vi "Move_to_Start.vi"(5 "Stop":refnum<vi>, 6 "Current Pos":refnum<vi>, 7 "Complete?":refnum<vi>, 8 "Move To":dbl, 9 "error in (no error)":errorcluster, 10 "MG17Motor":refnum<k7>(container)) -> (0 "error out":errorcluster, 2 "reference out":refnum<k7>)   [LabVIEW 2010]
panel:
  in  "#Turns":refnum<vi>
  out "Current":dbl
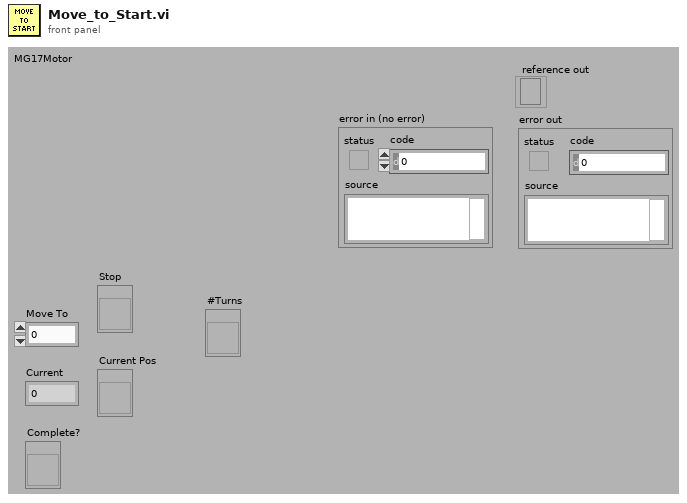
[diagram p1: front panel]
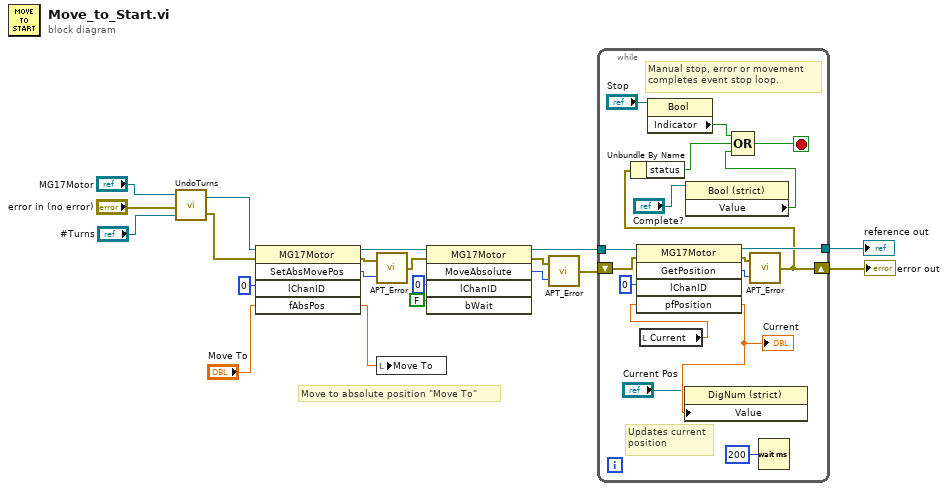
[diagram p0: block diagram]
diagram:
  # "Move to absolute position \"Move To\""
  n1 = call "UndoTurns.vi"("#Turns"="#Turns", "error in (no error)"="error in (no error)", "MG17Motor"="MG17Motor") -> ("error out"=w2:errorcluster, "MG17MotorOut"=w1:refnum<k7>)
  n2 = invoke class="MG17Motor" method="SetAbsMovePos"(reference=w1, error in=w2, "lChanID"=0, "fAbsPos"="Move To") -> (reference out=w6:refnum<k7>, error out=w15:errorcluster, "SetAbsMovePos"=w14:i32, "fAbsPos"=w18:sgl)  [unwired: 1 in, 1 out]
  n3 = call "APT_Error.vi"("Return Code"=w14, "error in (no error)"=w15) -> ("error out"=w13:errorcluster)
  n4 = local write "Move To"(w18) -> ()
  n5 = invoke class="MG17Motor" method="MoveAbsolute"(reference=w6, error in=w13, "lChanID"=0, "bWait"=FALSE) -> (reference out=w9:refnum<k7>, error out=w12:errorcluster, "MoveAbsolute"=w11:i32)  [unwired: 1 in, 2 out]
  n6 = call "APT_Error.vi"("Return Code"=w11, "error in (no error)"=w12) -> ("error out"=w10:errorcluster)
  n7 = while {
    shift-right: [w30] -> w8
    shift-left: w10 -> [w33]
    tunnel: w9 -> [w35]
    tunnel: [w34] -> w7
    stop <- w28 stop-if-true
    # "Updates current\nposition"
    # "Manual stop, error or movement\ncompletes event stop loop."
    n8 = local read "Current"() -> (w26:dbl)
    n9 = invoke class="MG17Motor" method="GetPosition"(reference=w35, error in=w33, "lChanID"=0, "pfPosition"=w26) -> (reference out=w34:refnum<k7>, error out=w37:errorcluster, "GetPosition"=w36:i32, "pfPosition"=w27:sgl)  [unwired: 1 in, 1 out]
    "Current" <- w27
    n10 = property class="Bool"(reference="Stop") -> ("Indicator"=w21:bool)  [unwired: 1 in, 2 out]
    n11 = property class="DigNum (strict)"(reference="Current Pos", "Value"=w27) -> ()  [unwired: 1 in, 2 out]
    n12 = property class="Bool (strict)"(reference="Complete?") -> ("Value"=w23:bool)  [unwired: 1 in, 2 out]
    n13 = call "APT_Error.vi"("Return Code"=w36, "error in (no error)"=w37) -> ("error out"=w30:errorcluster)
    n14 = Unbundle By Name(w30) -> ("status"=w29:bool)
    n15 = Compound Arithmetic op=OR(w21, w29, w23) -> (w28:bool)
    n16 = Wait (ms)(milliseconds to wait=u32 200) -> ()  [unwired: 1 out]
  }
  "reference out" <- w7
  "error out" <- w8
